vi "Zero Out Friction.vi"(8 "error in (no error)":errorcluster, 11 "serial arm in":refnum<class "NI_Robotics_Serial Robot Arm.lvclass">) -> (0 "error out":errorcluster, 3 "serial arm out":refnum<class "NI_Robotics_Serial Robot Arm.lvclass">)   [LabVIEW 2017, in "NI_Robotics_Serial Robot Arm.lvclass"]
doc: "Sets the amount of friction of every joint in <B>serial arm in</B> to 0.\n\n<B>.m file:</B> nofriction"
uses:
  <vilib>/robotics/Kinematics/Robot/NI_Robotics_Serial Robot Arm.lvclass
  <vilib>/robotics/Kinematics/Robot/NI_Robotics_Serial Robot Arm.lvclass/NI_Robotics_Serial Robot Arm.ctl
  <vilib>/robotics/Kinematics/Link/NI_Robotics_Link.lvclass
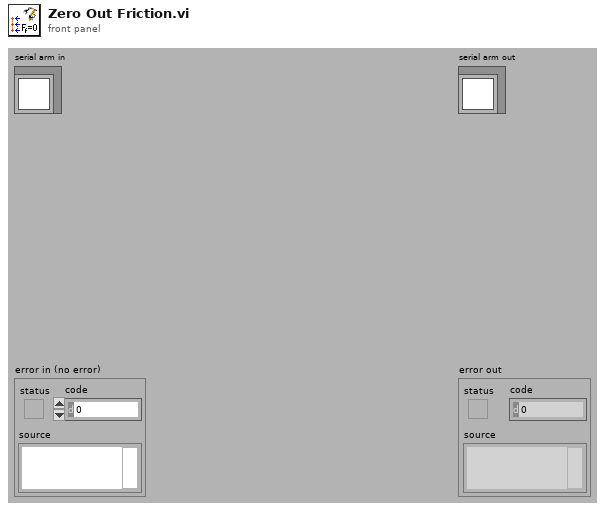
[diagram p1: front panel]
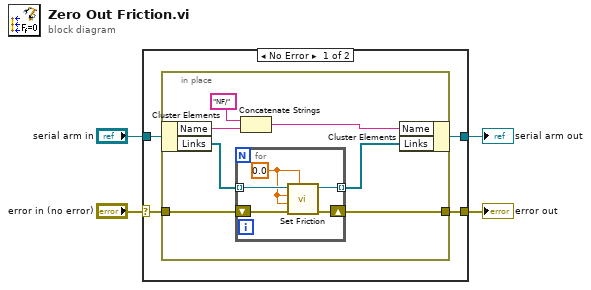
[diagram p0: block diagram]
diagram:
  n1 = case shown="No Error" "error in (no error)" {
    selector: "error in (no error)" -> [w6 w22]
    tunnel: [w5 w22] -> w3
    tunnel: [w7 w21] -> w1
    tunnel: "serial arm in" -> [w8 w21]
    frame No Error {
      n2 = in-place {
        in-place-border: w6 -> [w10]
        in-place-border: [w9] -> w5
        n3 = in-place-cluster #1(w8) -> ("Name"=w14:string, "Links"=w12:refnum<class "NI_Robotics_Link.lvclass">[])
        n4 = for {
          tunnel: w12 -> [w20] mode=indexing
          tunnel: [w19] -> w11 mode=indexing
          shift-right: [w16] -> w9
          shift-left: w10 -> [w17]
          w18 = 0.0 ("Positive Coulomb Friction")
          n5 = call <vilib>:"Set Friction.vi"("Viscous Friction"=w18, "error in (no error)"=w17, "Negative Coulomb Friction"=w18, "Positive Coulomb Friction"=w18, "Link in"=w20) -> ("error out"=w16:errorcluster, "Link out"=w19:refnum<class "NI_Robotics_Link.lvclass">)  [unwired: 5 in]
        }
        n6 = Concatenate Strings("NF/", w14) -> (w13:string)
        n7 = in-place-cluster #1("Name"=w13, "Links"=w11) -> (w7:refnum<class "NI_Robotics_Serial Robot Arm.lvclass">)
      }
    }
    frame Error {
    }
  }
  "error out" <- w3
  "serial arm out" <- w1
